vi "to string.vi"(8 "error in":errorcluster, 11 "EthernetIP configuration in":refnum<class "EthernetIP configuration.lvclass">) -> (0 "error out":errorcluster, 1 "data":string, 2 "version":string, 3 "EthernetIP configuration out":refnum<class "EthernetIP configuration.lvclass">)   [LabVIEW 2013, in "EthernetIP configuration.lvclass"]
doc: "Provides an interface for saving a module configuration to a file or other serialized data source. It is recommended that all children of this class store data in two sets--data required for its own initialization, and any data required for parent initialization--and that each implementation uses the <b>Call Parent Method</b> primitive to serialize parent information."
uses:
  EthernetIP configuration.lvclass
  <vilib>/NI/Tag Bus Module Framework/module configuration/TBM module configuration.lvclass
  EthernetIP configuration.lvclass/EthernetIP configuration.ctl
  <vilib>/NI/Tag Bus Module Framework/root configuration/unwrap data.vi
  current version.vi
  <vilib>/NI/Tag Bus Module Framework/root configuration/TBM configuration.lvclass
  channel/EthernetIP Channel.lvclass
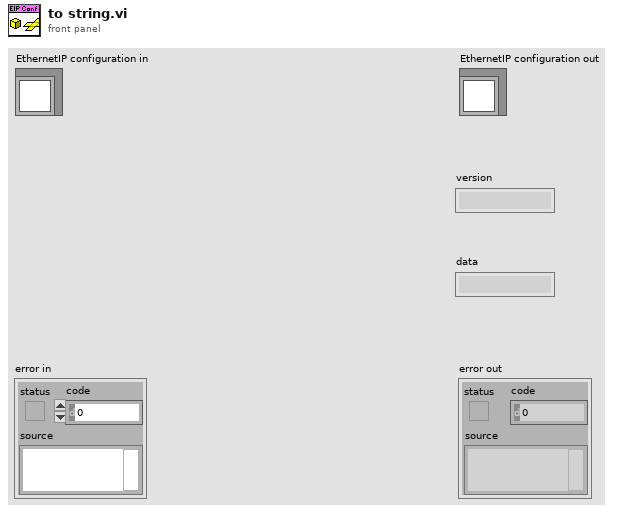
[diagram p1: front panel]
types:
  T1 = typedef "EthernetIP configuration.lvclass/assembly definition.ctl" = cluster{"name":string, "Instance ID":u32, "Type":T2, "Size (bytes)":u32}
  T2 = typedef "EthernetIP configuration.lvclass/assembly type.ctl" = enum32{"Producing", "Consuming"}
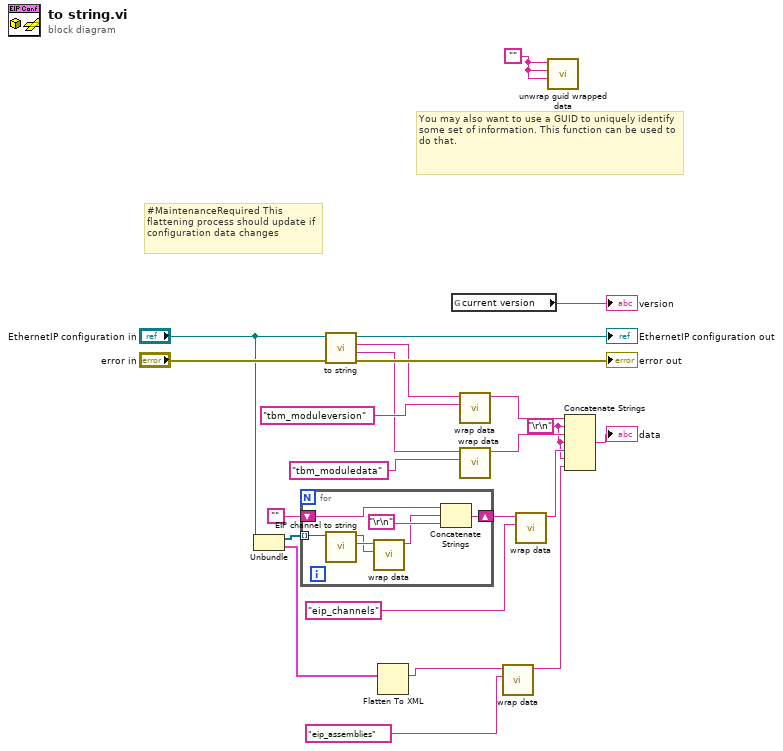
[diagram p0: block diagram]
diagram:
  w5 = "\r\n"
  w13 = ""
  # "You may also want to use a GUID to uniquely identify some set of information. This function can be used to do that."
  # "#MaintenanceRequired This flattening process should update if configuration data changes"
  n1 = Unbundle("EthernetIP configuration in") -> (w8:refnum<class "EthernetIP Channel.lvclass">[], w2:T1[])
  n2 = for {
    tunnel: w8 -> [w30] mode=indexing
    shift-right: [w26] -> w6
    shift-left: "" -> [w25]
    n3 = call "EIP channel to string.vi"("channel in"=w30) -> ("channel data"=w29:string, "identifier"=w28:string)  [unwired: 9 in]
    n4 = call <vilib>:"wrap data.vi"("identifier"=w28, "data to wrap"=w29) -> ("wrapped data"=w24:string)  [unwired: 9 in]
    n5 = Concatenate Strings(w25, w24, "\r\n") -> (w26:string)
  }
  n6 = call-parent "to string.vi"("error in"="error in", "module configuration in"="EthernetIP configuration in") -> ("error out"=→"error out":errorcluster, "data"=w14:string, "version"=w15:string, "module configuration out"=→"EthernetIP configuration out":refnum<class "EthernetIP configuration.lvclass">)  [unwired: 6 in]
  n7 = Flatten To XML(anything=w2) -> (xml string=w1:string)
  n8 = global read "current version.vi" "current version"() -> (→"version":string)
  n9 = call <vilib>:"wrap data.vi"("identifier"="tbm_moduleversion" ("additional identifier"), "data to wrap"=w15) -> ("wrapped data"=w17:string)  [unwired: 9 in]
  n10 = call <vilib>:"wrap data.vi"("identifier"="tbm_moduledata" ("additional identifier"), "data to wrap"=w14) -> ("wrapped data"=w16:string)  [unwired: 9 in]
  n11 = call <vilib>:"wrap data.vi"("identifier"="eip_assemblies" ("additional identifier"), "data to wrap"=w1) -> ("wrapped data"=w3:string)  [unwired: 9 in]
  n12 = call <vilib>:"wrap data.vi"("identifier"="eip_channels" ("additional identifier"), "data to wrap"=w6) -> ("wrapped data"=w10:string)  [unwired: 9 in]
  n13 = call <vilib>:"unwrap guid wrapped data.vi"("identifier"=w13, "uuid"=w13, "data to unwrap"=w13) -> ()  [unwired: 7 in, 2 out]
  n14 = Concatenate Strings(w17, w5, w16, w5, w10, w5, w3) -> (→"data":string)
